vi "DE_Crossover.vi"(6 "DE settings":T3={"population size"=10, "scale factor"=0.9, "crossover probability"=0.95, "bound mapping method"=1, "mutation method"=0, "crossover method"=0} {"crossover method" items=["Uniform", "Exponential"]; "mutation method" items=["Random", "Either Or", "Best", "Target to Best"]; "bound mapping method" items=["None", "Random between Bounds and Values", "Re-Initialize"]}, 8 "error in (no error)":errorcluster, 9 "State In":T1) -> (0 "error out":errorcluster, 1 "State Out":T1, 2 "Base Indexes":i32[](array[numeric]), 3 "Candidate State":T1)   [LabVIEW 2020, in "NI_AAL_GlobalOptimization.lvlib"]
uses:
  <vilib>/gmath/NI_AAL_GlobalOptimization.lvlib
  <vilib>/gmath/GlobalOptimization.llb/DE_State.ctl
  <vilib>/gmath/GlobalOptimization.llb/DE_Population.ctl
  <vilib>/gmath/GlobalOptimization.llb/DE_Settings.ctl
  <vilib>/gmath/GlobalOptimization.llb/DE_Bound Mapping Method.ctl
  <vilib>/gmath/GlobalOptimization.llb/DE_Mutation Method.ctl
  <vilib>/gmath/GlobalOptimization.llb/DE_Crossover Method.ctl
  <vilib>/Analysis/1siggen.llb/Riffle Array (I32).vi
  <vilib>/Analysis/NI_AALBase.lvlib
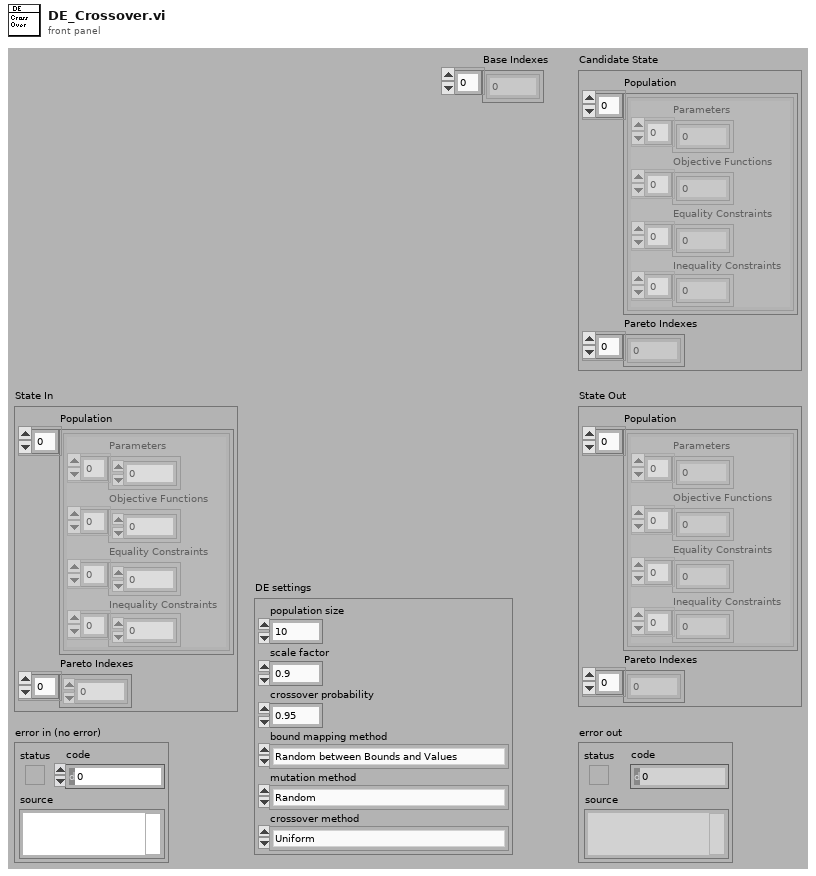
[diagram p1: front panel]
types:
  T1 = typedef "NI_AAL_GlobalOptimization.lvlib/DE_State.ctl" = cluster{"Population":T2[], "Pareto Indexes":i32[]}
  T2 = typedef "NI_AAL_GlobalOptimization.lvlib/DE_Population.ctl" = cluster{"Parameters":dbl[], "Objective Functions":dbl[], "Equality Constraints":dbl[], "Inequality Constraints":dbl[]}
  T3 = typedef "NI_AAL_GlobalOptimization.lvlib/DE_Settings.ctl" = cluster{"population size":i32, "scale factor":dbl, "crossover probability":dbl, "bound mapping method":T4, "mutation method":T5, "crossover method":T6}
  T4 = typedef "NI_AAL_GlobalOptimization.lvlib/DE_Bound Mapping Method.ctl" = u16
  T5 = typedef "NI_AAL_GlobalOptimization.lvlib/DE_Mutation Method.ctl" = u16
  T6 = typedef "NI_AAL_GlobalOptimization.lvlib/DE_Crossover Method.ctl" = u16
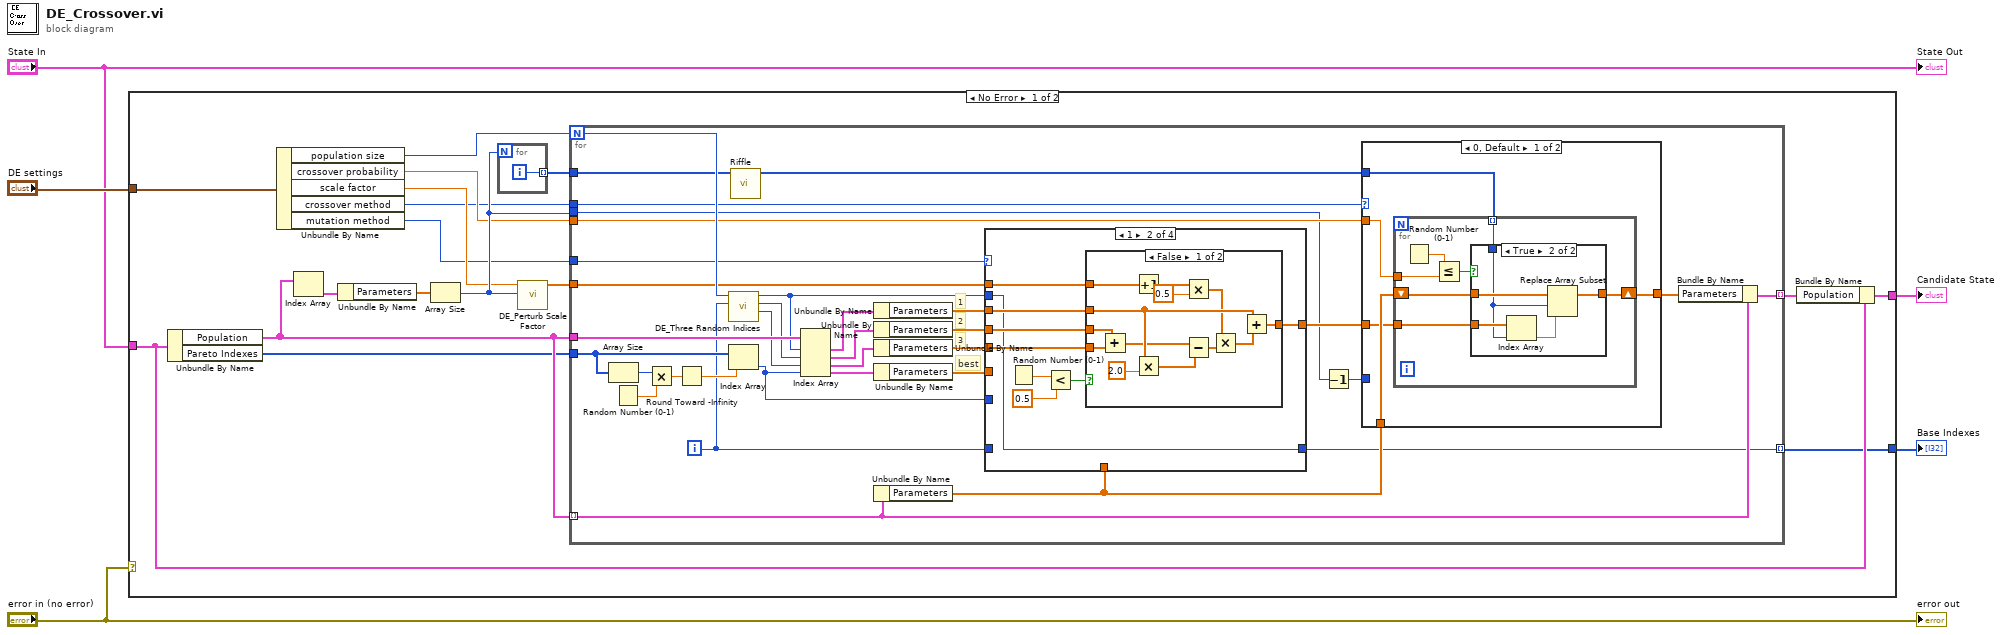
[diagram p0: block diagram]
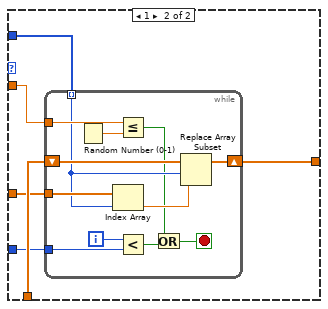
[diagram p3: hidden frame]
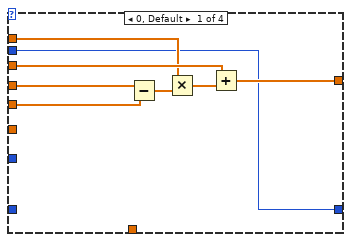
[diagram p4: hidden frame]
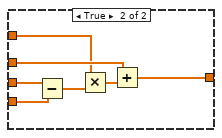
[diagram p5: hidden frame]
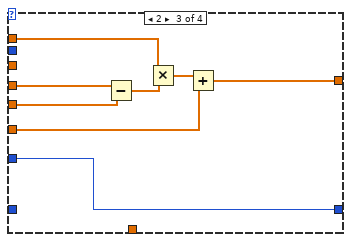
[diagram p6: hidden frame]
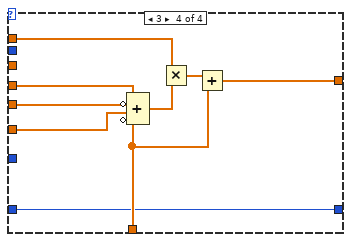
[diagram p7: hidden frame]
diagram:
  n1 = case shown="No Error" "error in (no error)" {
    tunnel: "DE settings" -> [w21 _]
    tunnel: "State In" -> [w9 w148]
    tunnel: [w8 w148] -> w3
    tunnel: [w6 _] -> w1
    frame No Error {
      n2 = Unbundle By Name(w9) -> ("Population"=w11:T2[], "Pareto Indexes"=w10:i32[])
      n3 = Unbundle By Name(w21) -> ("population size"=w17:i32, "crossover probability"=w16:dbl, "scale factor"=w14:dbl, "crossover method"=w13:T6, "mutation method"=w7:T5)
      n4 = Index Array(array=w11) -> (element=w20:T2)  [unwired: 1 in]
      n5 = Unbundle By Name(w20) -> ("Parameters"=w19:dbl[])
      n6 = Array Size(array=w19) -> (size(s)=w18:i32)
      n7 = for {
        N: w18 -> [_]
        tunnel: [w23] -> w22 mode=indexing
        i -> [w23]
      }
      n8 = call <vilib>:"DE_Perturb Scale Factor.vi"("number of parameters"=w18, "scale factor"=w14) -> ("Perturbed Scale Factors"=w15:dbl[])  [unwired: 9 in]
      n9 = for {
        N: w17 -> [w46]
        tunnel: w11 -> [w57]
        tunnel: w16 -> [w43]
        tunnel: w11 -> [w48] mode=indexing
        tunnel: [w47] -> w12 mode=indexing
        tunnel: w15 -> [w45]
        tunnel: w22 -> [w25]
        tunnel: w7 -> [w42]
        tunnel: w13 -> [w41]
        tunnel: w18 -> [w40]
        tunnel: w10 -> [w33]
        tunnel: [w26] -> w6 mode=indexing
        i -> [w29]
        # "best"
        # "3"
        # "2"
        # "1"
        n10 = Array Size(array=w33) -> (size(s)=w37:i32)
        n11 = Random Number (0-1)() -> (number: 0 to 1=w36:dbl)
        n12 = Multiply(x=w37, y=w36) -> (x*y=w35:dbl)
        n13 = Round Toward -Infinity(1:w35) -> (0:w34:dbl)
        n14 = call <vilib>:"DE_Three Random Indices.vi"("cur index"=w29, "population size"=w46) -> ("index 2"=w55:i32, "index 1"=w56:i32, "index 0"=w28:i32)  [unwired: 7 in]
        n15 = Index Array(array=w33, index=w34) -> (element=w27:i32)
        n16 = call-poly <vilib>:"Riffle.vi"("X"=w25) -> ("Riffled {X}"=w24:i32[])  [unwired: 8 in, 2 out]
        n17 = Index Array(array=w57, index #1=w28, index #2=w56, index #3=w55, index #4=w27) -> (element #1=w54:T2, element #2=w53:T2, element #3=w52:T2, element #4=w32:T2)
        n18 = Unbundle By Name(w54) -> ("Parameters"=w51:dbl[])
        n19 = Unbundle By Name(w53) -> ("Parameters"=w50:dbl[])
        n20 = Unbundle By Name(w52) -> ("Parameters"=w49:dbl[])
        n21 = Unbundle By Name(w32) -> ("Parameters"=w31:dbl[])
        n22 = Unbundle By Name(w48) -> ("Parameters"=w30:dbl[])
        n23 = case shown="1" w42 {
          tunnel: w51 -> [w101 w110 _ _]
          tunnel: w50 -> [w100 w109 w138 w147]
          tunnel: w49 -> [w99 w108 w137 w146]
          tunnel: w45 -> [w98 w107 w136 w145]
          tunnel: [w97 w106 w135 w144] -> w44
          tunnel: w31 -> [_ _ w132 w142]
          tunnel: w30 -> [_ _ _ w141]
          tunnel: w29 -> [_ _ _ w139]
          tunnel: [w94 w103 w131 w139] -> w26
          tunnel: w28 -> [w94 w103 _ _]
          tunnel: w27 -> [_ _ w131 _]
          frame 0, Default {
            n24 = Subtract(x=w100, y=w99) -> (x-y=w96:dbl[])
            n25 = Multiply(x=w98, y=w96) -> (x*y=w95:dbl[])
            n26 = Add(x=w101, y=w95) -> (x+y=w97:dbl[])
          }
          frame 1 {
            n27 = Random Number (0-1)() -> (number: 0 to 1=w105:dbl)
            n28 = Less?(x=w105, y=0.5) -> (x < y?=w104:bool)
            n29 = case shown="False" w104 {
              tunnel: w110 -> [w119 w130]
              tunnel: w109 -> [w121 w129]
              tunnel: w108 -> [w120 w128]
              tunnel: w107 -> [w123 w124]
              tunnel: [w113 w127] -> w106
              frame False {
                n30 = Add(x=w121, y=w120) -> (x+y=w118:dbl[])
                n31 = Increment(x=w123) -> (x+1=w122:dbl[])
                n32 = Multiply(x=w119, y=2.0) -> (x*y=w117:dbl[])
                n33 = Multiply(x=w122, y=0.5) -> (x*y=w115:dbl[])
                n34 = Subtract(x=w118, y=w117) -> (x-y=w116:dbl[])
                n35 = Multiply(x=w115, y=w116) -> (x*y=w114:dbl[])
                n36 = Add(x=w119, y=w114) -> (x+y=w113:dbl[])
              }
              frame True {
                n37 = Subtract(x=w129, y=w128) -> (x-y=w126:dbl[])
                n38 = Multiply(x=w124, y=w126) -> (x*y=w125:dbl[])
                n39 = Add(x=w130, y=w125) -> (x+y=w127:dbl[])
              }
            }
          }
          frame 2 {
            n40 = Subtract(x=w138, y=w137) -> (x-y=w134:dbl[])
            n41 = Multiply(x=w136, y=w134) -> (x*y=w133:dbl[])
            n42 = Add(x=w133, y=w132) -> (x+y=w135:dbl[])
          }
          frame 3 {
            n43 = Compound Arithmetic op=ADD(w147, invert w146, w142, invert w141) -> (w143:dbl[])
            n44 = Multiply(x=w145, y=w143) -> (x*y=w140:dbl[])
            n45 = Add(x=w140, y=w141) -> (x+y=w144:dbl[])
          }
        }
        n46 = Decrement(x=w40) -> (x-1=w39:i32)
        n47 = case shown="0, Default" w41 {
          tunnel: w24 -> [w62 w81]
          tunnel: w30 -> [w61 w80]
          tunnel: w44 -> [w60 w79]
          tunnel: w43 -> [w59 w78]
          tunnel: w39 -> [_ w77]
          tunnel: [w58 w76] -> w38
          frame 0, Default {
            n48 = for {
              tunnel: w62 -> [w65] mode=indexing
              tunnel: w60 -> [w66]
              tunnel: w59 -> [w68]
              shift-right: [w64] -> w58
              shift-left: w61 -> [w67]
              n49 = Random Number (0-1)() -> (number: 0 to 1=w69:dbl)
              n50 = Less Or Equal?(x=w69, y=w68) -> (x <= y?=w63:bool)
              n51 = case shown="True" w63 {
                tunnel: w67 -> [w70 w75]
                tunnel: w66 -> [_ w74]
                tunnel: w65 -> [_ w73]
                tunnel: [w70 w71] -> w64
                frame False {
                }
                frame True {
                  n52 = Index Array(array=w74, index=w73) -> (element=w72:dbl)
                  n53 = Replace Array Subset(array=w75, new element=w72, index=w73) -> (w71:dbl[])
                }
              }
            }
          }
          frame 1 {
            n54 = while {
              tunnel: w81 -> [w89] mode=indexing
              tunnel: w79 -> [w90]
              tunnel: w78 -> [w92]
              shift-right: [w87] -> w76
              shift-left: w80 -> [w91]
              tunnel: w77 -> [w85]
              i -> [w86]
              stop <- w82 stop-if-true
              n55 = Random Number (0-1)() -> (number: 0 to 1=w93:dbl)
              n56 = Index Array(array=w90, index=w89) -> (element=w88:dbl)
              n57 = Less Or Equal?(x=w92, y=w93) -> (x <= y?=w83:bool)
              n58 = Less?(x=w86, y=w85) -> (x < y?=w84:bool)
              n59 = Or(x=w83, y=w84) -> (x .or. y?=w82:bool)
              n60 = Replace Array Subset(array=w91, new element=w88, index=w89) -> (w87:dbl[])
            }
          }
        }
        n61 = Bundle By Name(cluster=w48, "Parameters"=w38) -> (w47:T2)
      }
      n62 = Bundle By Name(cluster=w9, "Population"=w12) -> (w8:T1)
    }
    frame Error {
    }
  }
  "Candidate State" <- w3
  "Base Indexes" <- w1
  "State Out" <- "State In"
  "error out" <- "error in (no error)"
